vi "hardware_apply_settings.vi"(8 "error in (no error)":errorcluster, 11 "newport_xps in":refnum<class "newport_xps.lvclass">) -> (0 "error out":errorcluster, 3 "newport_xps out":refnum<class "newport_xps.lvclass">)   [LabVIEW 2015, in "newport_xps.lvclass"]
uses:
  newport_xps.lvclass
  newport_xps.lvclass/newport_xps.ctl
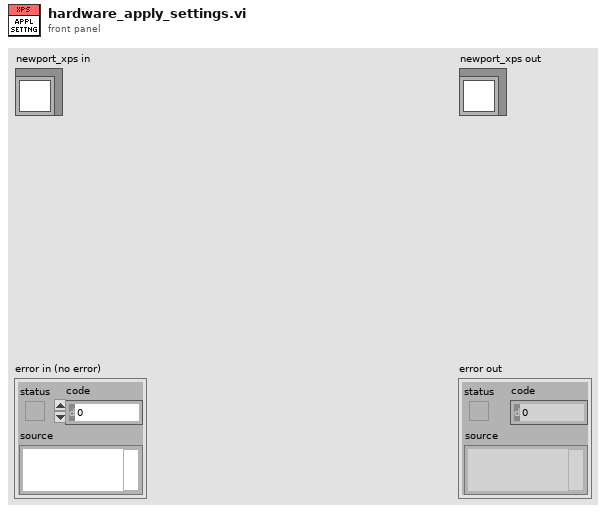
[diagram p1: front panel]
types:
  T1 = cluster{"connection TCP":refnum<k5>, "LogTo File":bool, "Log File refnum":refnum<file>, "no error if error log":bool}
  T2 = cluster{"Velocity (units/seconds)":dbl, "Acceleration (units/seconds²)":dbl, "Minimum Jerk Time (seconds)":dbl, "Maximum Jerk Time (seconds)":dbl}
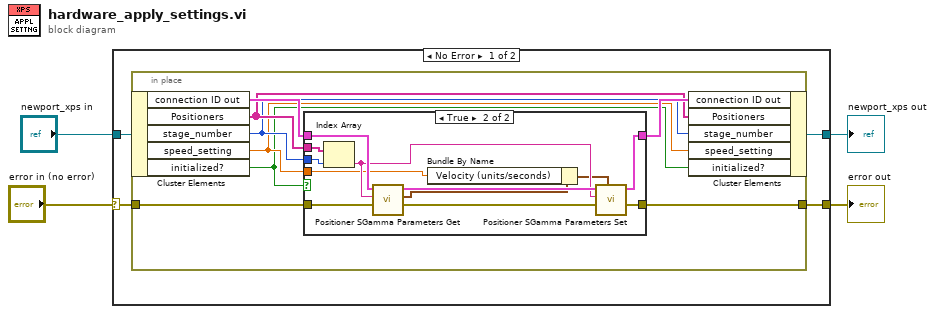
[diagram p0: block diagram]
diagram:
  n1 = case shown="No Error" "error in (no error)" {
    selector: "error in (no error)" -> [w7 w32]
    tunnel: "newport_xps in" -> [w8 w31]
    tunnel: [w6 w31] -> w2
    tunnel: [w5 w32] -> w1
    frame No Error {
      n2 = in-place {
        in-place-border: w7 -> [w15]
        in-place-border: [w13] -> w5
        n3 = in-place-cluster #1(w8) -> ("connection ID out"=w14:T1, "Positioners"=w12:string[], "stage_number"=w11:i32, "speed_setting"=w10:dbl, "initialized?"=w9:bool)
        n4 = case shown="True" w9 {
          tunnel: [w18 w30] -> w16
          tunnel: w15 -> [w17 w29]
          tunnel: w14 -> [w18 w27]
          tunnel: [w17 w22] -> w13
          tunnel: w12 -> [_ w21]
          tunnel: w11 -> [_ w20]
          tunnel: w10 -> [_ w19]
          frame False {
          }
          frame True {
            n5 = Index Array(array=w21, index=w20) -> (element=w25:string)
            n6 = call "Positioner SGamma Parameters Get.vi"("XPS error in (no error)"=w29, "Positioner Name (250 c max)"=w25, "connection ID in"=w27) -> ("XPS error out"=w28:errorcluster, "SGamma Parameters"=w24:T2, "connection ID out"=w26:T1)  [unwired: 5 in, 1 out]
            n7 = Bundle By Name(cluster=w24, "Velocity (units/seconds)"=w19) -> (w23:T2)
            n8 = call "Positioner SGamma Parameters Set.vi"("SGamma Parameters"=w23, "XPS error in (no error)"=w28, "Positioner Name (250 c max)"=w25, "connection ID in"=w26) -> ("XPS error out"=w22:errorcluster, "connection ID out"=w30:T1)  [unwired: 5 in, 1 out]
          }
        }
        n9 = in-place-cluster #1("connection ID out"=w16, "Positioners"=w12, "stage_number"=w11, "speed_setting"=w10, "initialized?"=w9) -> (w6:refnum<class "newport_xps.lvclass">)
      }
    }
    frame Error {
    }
  }
  "error out" <- w1
  "newport_xps out" <- w2
